vi "LeakageSensor.vi"(2 "error in (no error)":errorcluster) -> (0 "error out":errorcluster, 1 "WarningLIGHT":bool)   [LabVIEW 2013]
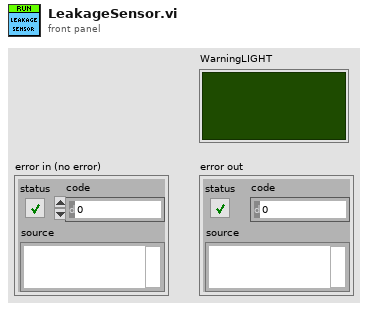
[diagram p1: front panel]
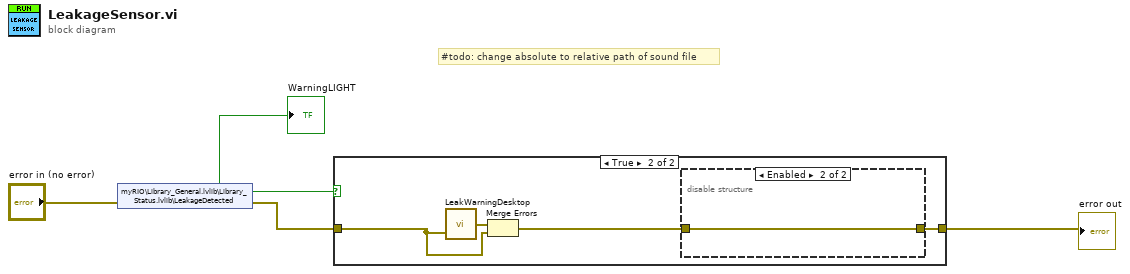
[diagram p0: block diagram]
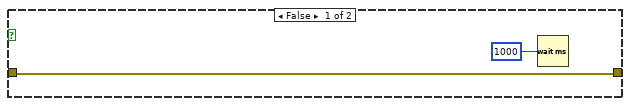
[diagram p2: hidden frame]
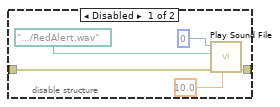
[diagram p3: hidden frame]
diagram:
  # "#todo: change absolute to relative path of sound file"
  n1 = shared-variable "myRIO\\Library_General.lvlib\\Library_Status.lvlib\\LeakageDetected"(error in="error in (no error)") -> (w3:bool, error out=w4:errorcluster)
  "WarningLIGHT" <- w3
  n2 = case shown="True" w3 {
    tunnel: w4 -> [w5 w8]
    tunnel: [w5 w10] -> w1
    frame False {
      n3 = Wait (ms)(milliseconds to wait=u32 1000) -> ()  [unwired: 1 out]
    }
    frame True {
      n4 = call "LeakWarningDesktop.vi"("error in (no error)"=w8) -> ("error out"=w9:errorcluster)  [unwired: 1 in]
      n5 = Merge Errors(w9, w8) -> (w7:errorcluster)
      n6 = disable-structure shown="Enabled" {
        disable-tunnel: [w12 w16] -> w10
        disable-tunnel: w7 -> [w11 w16]
        frame Disabled {
          n7 = call <vilib>:"Play Sound File.vi"("timeout (sec)"=10.0, "error in (no error)"=w11, "path"=path ".../RedAlert.wav", "device ID"=u32 0) -> ("error out"=w12:errorcluster)  [unwired: 6 in, 1 out]
        }
        frame Enabled {
        }
      }
    }
  }
  "error out" <- w1
